vi "GetPhraseForPhraseLowLevel.vi"(7 "Dictionary":T1, 8 "error in (no error)":errorcluster, 10 "Target Language":string, 11 "Phrase":string) -> (0 "error out":errorcluster, 3 "Phrase In Target Language":string)   [LabVIEW 2020]
uses:
  Dictionary--Cluster.ctl
  Font -- Cluster.ctl
  Phrase Dictionary Entry -- Cluster.ctl
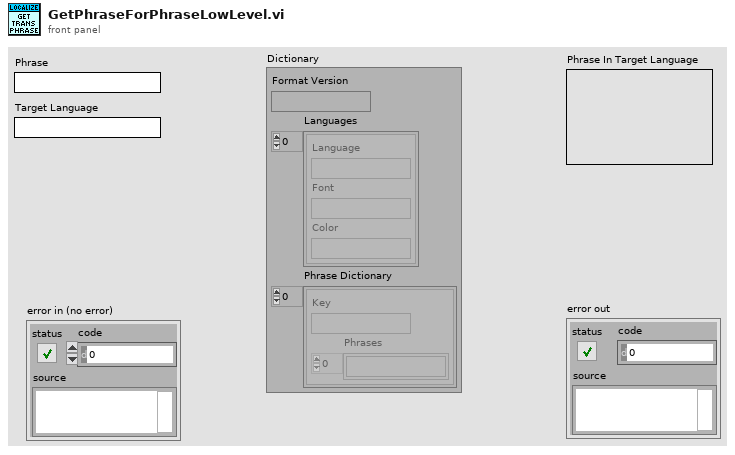
[diagram p1: front panel]
types:
  T1 = typedef "Dictionary--Cluster.ctl" = cluster{"Format Version":string, "Languages":T2[], "Phrase Dictionary":T3[]}
  T2 = typedef "Font -- Cluster.ctl" = cluster{"Language":string, "Font":string, "Color":string}
  T3 = typedef "Phrase Dictionary Entry -- Cluster.ctl" = cluster{"Key":string, "Phrases":string[]}
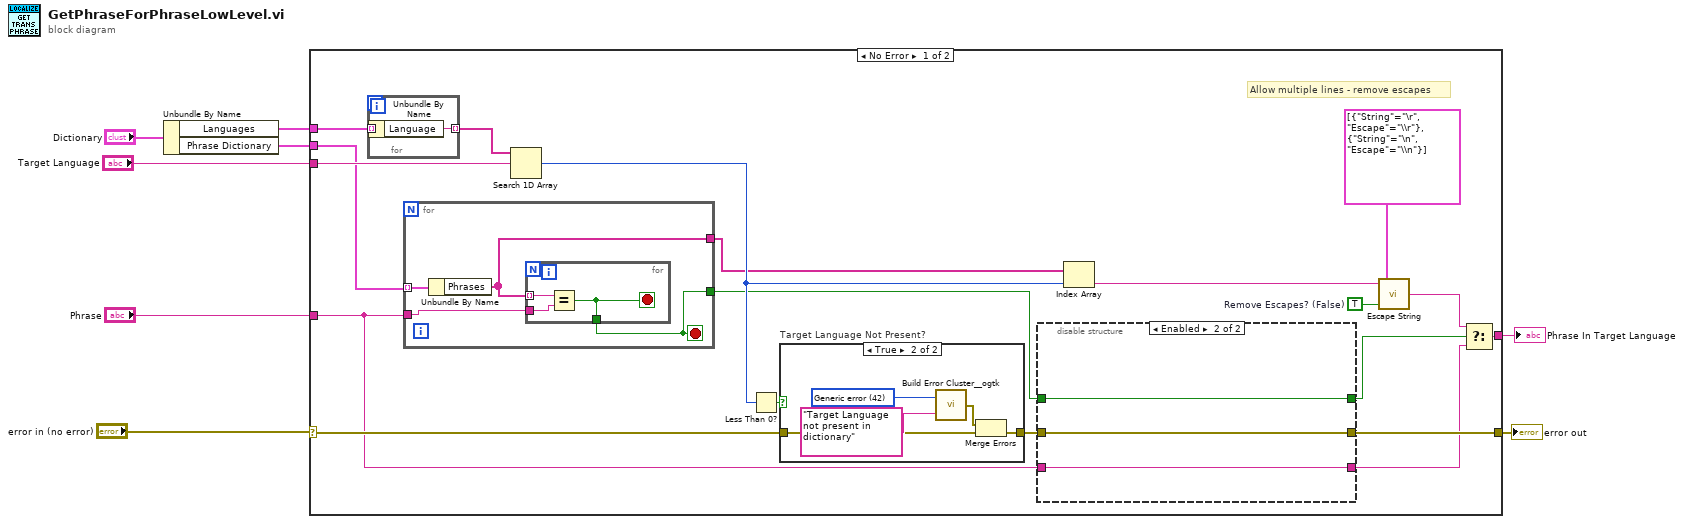
[diagram p0: block diagram]
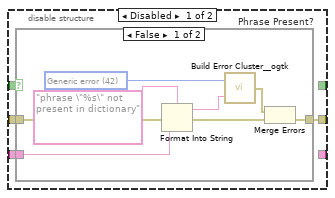
[diagram p2: hidden frame]
diagram:
  n1 = Unbundle By Name("Dictionary") -> ("Languages"=w3:T2[], "Phrase Dictionary"=w1:T3[])
  n2 = case shown="No Error" "error in (no error)" {
    selector: "error in (no error)" -> [w23 w59]
    tunnel: w3 -> [w17 _]
    tunnel: [w18 _] -> w8
    tunnel: [w19 w59] -> w7
    tunnel: "Target Language" -> [w22 _]
    tunnel: "Phrase" -> [w14 _]
    tunnel: w1 -> [w15 _]
    frame No Error {
      w25 = TRUE  # Remove Escapes? (False)
      # "Allow multiple lines - remove escapes"
      n3 = for {
        tunnel: w17 -> [w52] mode=indexing
        tunnel: [w51] -> w16 mode=indexing
        n4 = Unbundle By Name(w52) -> ("Language"=w51:string)
      }
      n5 = for {
        tunnel: w15 -> [w47] mode=indexing
        tunnel: w14 -> [w45]
        tunnel: [w46] -> w12
        tunnel: [w44] -> w13
        stop <- w46 stop-if-true
        n6 = Unbundle By Name(w47) -> ("Phrases"=w44:string[])
        n7 = for {
          tunnel: [w50] -> w46
          tunnel: w44 -> [w49] mode=indexing
          tunnel: w45 -> [w48]
          stop <- w50 stop-if-true
          n8 = Equal?(x=w49, y=w48) -> (x = y?=w50:bool)
        }
      }
      n9 = Search 1D Array(1D array=w16, element=w22) -> (index of element=w21:i32)  [unwired: 1 in]
      n10 = Less Than 0?(x=w21) -> (x < 0?=w27:bool)
      n11 = case "Target Language Not Present?" shown="True" w27 {
        tunnel: w23 -> [w53 w55]
        tunnel: [w53 w54] -> w26
        frame False {
        }
        frame True {
          w58 = 42 items=["No error", "Argument error", "Memory is full", "Out of zone", "End of file", "File already open", "Generic file I/O error", "File not found", "File permission error", "Disk is full", "Duplicate path", "Too many files open", "System feature not enabled", "Resource file not found", "Cannot add resource", "Resource not found", "Image not found", "Image memory error", "Pen does not exist", "Config type invalid", "Config token not found", "Config parse error", "Config memory error", "Bad external code format", "Bad external code offset", "External code not present", "Null window", "Destroy window error", "Null menu", "Print aborted", "Bad print record", "Print driver error", "Windows error during printing", "Memory error during printing", "Print dialog error", "Generic print error", "Invalid device refnum", "Device not found", "Device parameter error", "Device unit error", "Cannot open device", "Device call aborted", "Generic error", "Cancelled by user", "Object ID too low", "Object ID too high", "Object not in heap", "Unknown heap", "Unknown object (invalid DefProc)", "Unknown object (DefProc not in table)", "Message out of range", "Invalid (null) method", "Unknown message", "Manager call not supported", "Bad address", "Network operation in progress", "Network operation timed out", "Connection is busy", "Network attribute not supported", "Network error", "Address in use", "System out of memory", "Connection aborted", "Connection refused", "Not connected", "Already connected", "Connection closed", "Initialization error (interapplication manager)", "Bad occurrence", "Wait on unbound occurrence handler", "Occurrence queue overflow", "Datalog type conflict", "Unused", "Unrecognized type (interapplication manager)", "Memory corrupt", "Failed to make temporary DLL", "Old CIN version", "Drag socket not found", "Failed to load drop-object", "Failed to register OLE object", "Failed to release OLE object", "Format specifier type mismatch", "Unknown format specifier", "Too few format specifiers", "Too many format specifiers", "Scan failed", "Newer CIN version", "Error converting to variant", "Runtime menu error", "Password tampered", "Variant attribute not found", "Incompatible variant data type", "Event data is not available", "Event Store is not present", "Occurrence is not found", "Event Queue is not created", "Event info is not available", "Refnum passed is NULL", "Error retrieving Class GUID", "Error retrieving CoClass GUID", "Error retrieving TypeLib GUID.", "Bad built application magic bytes.", "Specific driver is different from the specific driver associated with the Logical Name.", "There is no session opened to the class driver.", "Max Error", "MAX - Error with config objects", "MAX - Error loading configuration", "MAX - Group not supported"]
          n12 = call <userlib>:"Build Error Cluster__ogtk.vi"("String to Prepend to source (\"\")"="Target Language not present in dictionary" ("String to Prepend to source (\"\")"), "code"=w58) -> ("error out"=w56:errorcluster)
          n13 = Merge Errors(w56, w55) -> (w54:errorcluster)
        }
      }
      n14 = disable-structure shown="Enabled" {
        disable-tunnel: w26 -> [w31 w43]
        disable-tunnel: [w30 w43] -> w19
        disable-tunnel: w14 -> [w29 w41]
        disable-tunnel: w12 -> [w28 w42]
        disable-tunnel: [_ w42] -> w10
        disable-tunnel: [_ w41] -> w9
        frame Disabled {
          n15 = case "Phrase Present?" shown="False" w28 {
            tunnel: w31 -> [w36 w40]
            tunnel: [w37 w40] -> w30
            tunnel: w29 -> [w33 _]
            frame False {
              w39 = 42 items=["No error", "Argument error", "Memory is full", "Out of zone", "End of file", "File already open", "Generic file I/O error", "File not found", "File permission error", "Disk is full", "Duplicate path", "Too many files open", "System feature not enabled", "Resource file not found", "Cannot add resource", "Resource not found", "Image not found", "Image memory error", "Pen does not exist", "Config type invalid", "Config token not found", "Config parse error", "Config memory error", "Bad external code format", "Bad external code offset", "External code not present", "Null window", "Destroy window error", "Null menu", "Print aborted", "Bad print record", "Print driver error", "Windows error during printing", "Memory error during printing", "Print dialog error", "Generic print error", "Invalid device refnum", "Device not found", "Device parameter error", "Device unit error", "Cannot open device", "Device call aborted", "Generic error", "Cancelled by user", "Object ID too low", "Object ID too high", "Object not in heap", "Unknown heap", "Unknown object (invalid DefProc)", "Unknown object (DefProc not in table)", "Message out of range", "Invalid (null) method", "Unknown message", "Manager call not supported", "Bad address", "Network operation in progress", "Network operation timed out", "Connection is busy", "Network attribute not supported", "Network error", "Address in use", "System out of memory", "Connection aborted", "Connection refused", "Not connected", "Already connected", "Connection closed", "Initialization error (interapplication manager)", "Bad occurrence", "Wait on unbound occurrence handler", "Occurrence queue overflow", "Datalog type conflict", "Unused", "Unrecognized type (interapplication manager)", "Memory corrupt", "Failed to make temporary DLL", "Old CIN version", "Drag socket not found", "Failed to load drop-object", "Failed to register OLE object", "Failed to release OLE object", "Format specifier type mismatch", "Unknown format specifier", "Too few format specifiers", "Too many format specifiers", "Scan failed", "Newer CIN version", "Error converting to variant", "Runtime menu error", "Password tampered", "Variant attribute not found", "Incompatible variant data type", "Event data is not available", "Event Store is not present", "Occurrence is not found", "Event Queue is not created", "Event info is not available", "Refnum passed is NULL", "Error retrieving Class GUID", "Error retrieving CoClass GUID", "Error retrieving TypeLib GUID.", "Bad built application magic bytes.", "Specific driver is different from the specific driver associated with the Logical Name.", "There is no session opened to the class driver.", "Max Error", "MAX - Error with config objects", "MAX - Error loading configuration", "MAX - Group not supported"]
              n16 = Format Into String(format string="phrase \"%s\" not present in dictionary" ("String to Prepend to source (\"\")"), error in=w36, w33) -> (resulting string=w32:string, error out=w35:errorcluster)  [unwired: 1 in]
              n17 = call <userlib>:"Build Error Cluster__ogtk.vi"("String to Prepend to source (\"\")"=w32, "code"=w39) -> ("error out"=w38:errorcluster)
              n18 = Merge Errors(w38, w35) -> (w37:errorcluster)
            }
            frame True {
            }
          }
        }
        frame Enabled {
        }
      }
      n19 = Index Array(array=w13, index=w21) -> (element=w20:string)
      n20 = call <vilib>:"Escape String.vi"("Remove Escapes? (False)"=w25, "Escapes"=cluster{"String":string, "Escape":string}[] [{"String"="\r", "Escape"="\\r"}, {"String"="\n", "Escape"="\\n"}], "String in"=w20) -> ("String out"=w11:string)
      n21 = Select(t=w11, s=w10, f=w9) -> (s? t:f=w18:string)
    }
    frame Error {
    }
  }
  "Phrase In Target Language" <- w8
  "error out" <- w7
